vi "Assignment_01_2.vi"() -> ()   [LabVIEW 2023]
uses:
  Operations.ctl
panel:
  out "C":i64
  in  "Operations":T1
  in  "Stop":bool
  in  "N":i64
  in  "M":i64
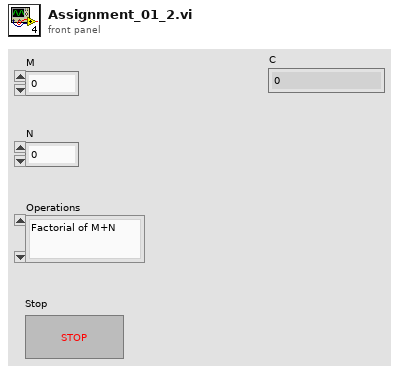
[diagram p1: front panel]
types:
  T1 = typedef "Operations.ctl" = enum16{"Factorial of M+N", "Sum of Factorial of first M Natural Numbers ", "Sum of Factorial of first N whole Numbers ", "Greater of M and N"}
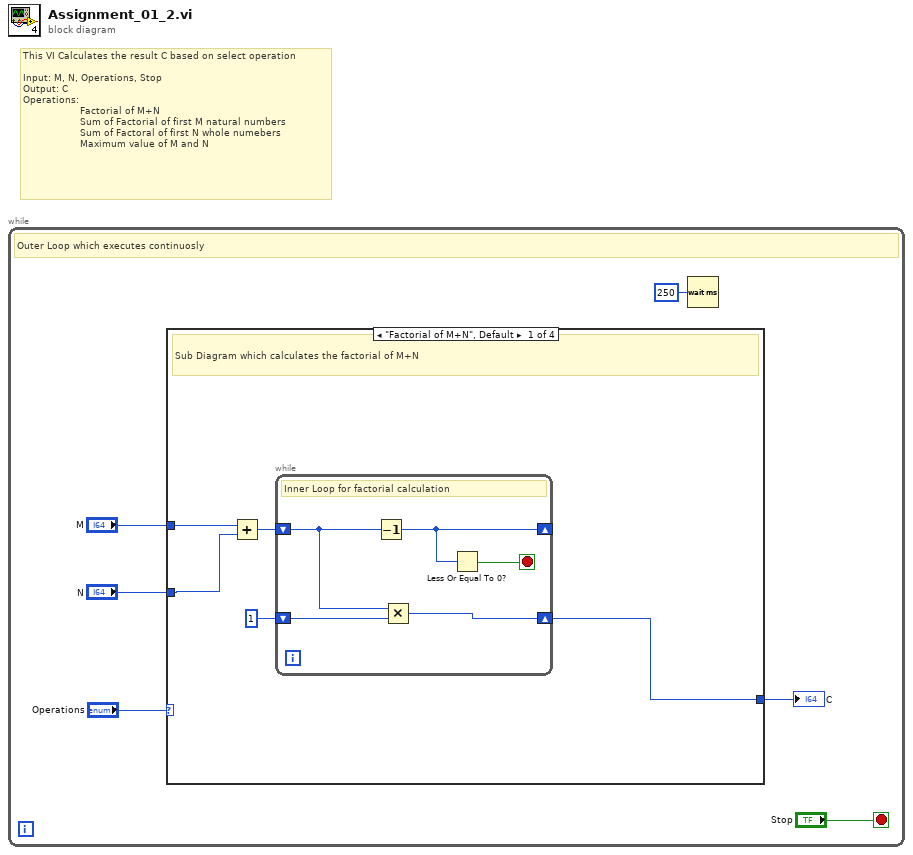
[diagram p0: block diagram]
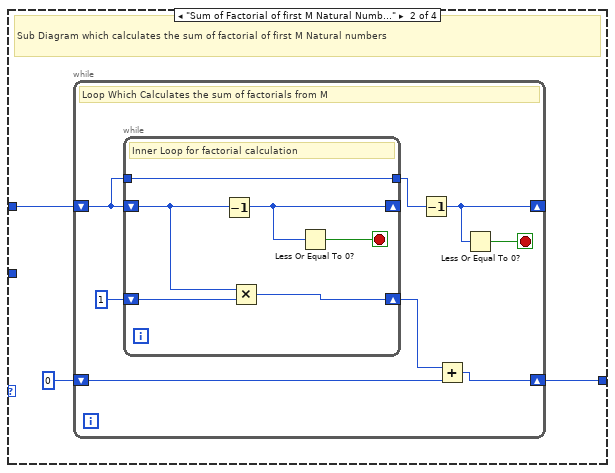
[diagram p2: hidden frame]
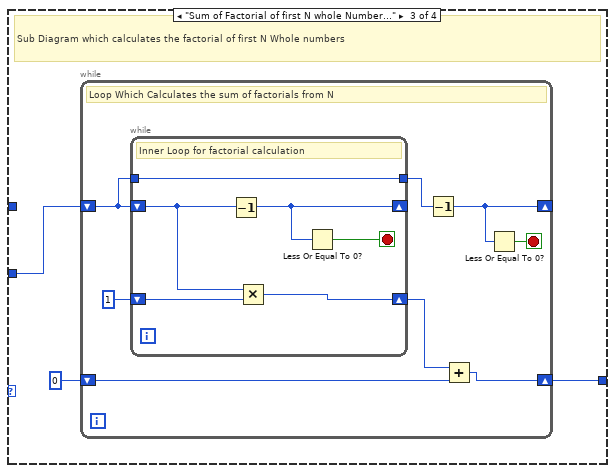
[diagram p3: hidden frame]
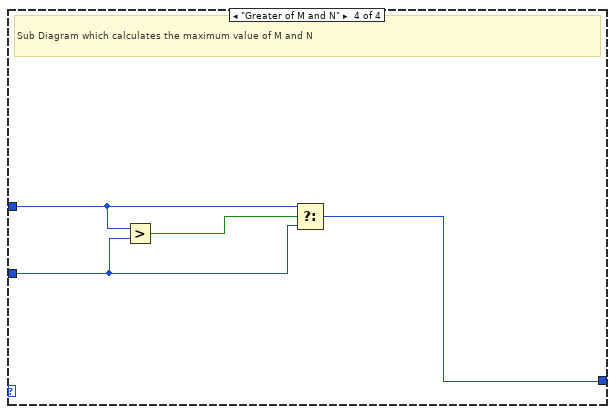
[diagram p4: hidden frame]
diagram:
  # "This VI Calculates the result C based on select operation\n\nInput: M, N, Operations, Stop\nOutput: C\nOperations:\n                   Factorial of M+N\n                   Sum of Factorial of first M natural numbers\n                   Sum of Factoral of first N whole numebers\n                   Maximum value of M and N"
  n1 = while {
    stop <- "Stop" stop-if-true
    # "Outer Loop which executes continuosly"
    n2 = case shown="\"Factorial of M+N\", Default" "Operations" {
      tunnel: "M" -> [w9 w19 _ w53]
      tunnel: "N" -> [w8 _ w35 w52]
      tunnel: [w7 w17 w34 w51] -> w3
      frame "Factorial of M+N", Default {
        # "Sub Diagram which calculates the factorial of M+N"
        n3 = Add(x=w9, y=w8) -> (x+y=w11:i64)
        n4 = while {
          shift-right: [w15] -> _
          shift-left: w11 -> [w12]
          shift-right: [w16] -> w7
          shift-left: i64 1 -> [w13]
          stop <- w14 stop-if-true
          # "Inner Loop for factorial calculation"
          n5 = Decrement(x=w12) -> (x-1=w15:i64)
          n6 = Multiply(x=w12, y=w13) -> (x*y=w16:i64)
          n7 = Less Or Equal To 0?(x=w15) -> (x <= 0?=w14:bool)
        }
      }
      frame "Sum of Factorial of first M Natural Numbers " {
        # "Sub Diagram which calculates the sum of factorial of first M Natural numbers"
        n8 = while {
          shift-right: [w25] -> _
          shift-left: w19 -> [w21]
          shift-right: [w22] -> w17
          shift-left: i64 0 -> [w24]
          stop <- w26 stop-if-true
          # "Loop Which Calculates the sum of factorials from M"
          n9 = while {
            shift-right: [w28] -> _
            shift-left: w21 -> [w31]
            shift-right: [w33] -> w23
            shift-left: i64 1 -> [w30]
            tunnel: [w29] -> w20
            tunnel: w21 -> [w29]
            stop <- w32 stop-if-true
            # "Inner Loop for factorial calculation"
            n10 = Decrement(x=w31) -> (x-1=w28:i64)
            n11 = Multiply(x=w31, y=w30) -> (x*y=w33:i64)
            n12 = Less Or Equal To 0?(x=w28) -> (x <= 0?=w32:bool)
          }
          n13 = Decrement(x=w20) -> (x-1=w25:i64)
          n14 = Add(x=w23, y=w24) -> (x+y=w22:i64)
          n15 = Less Or Equal To 0?(x=w25) -> (x <= 0?=w26:bool)
        }
      }
      frame "Sum of Factorial of first N whole Numbers " {
        # "Sub Diagram which calculates the factorial of first N Whole numbers"
        n16 = while {
          shift-right: [w42] -> _
          shift-left: w35 -> [w38]
          shift-right: [w39] -> w34
          shift-left: i64 0 -> [w41]
          stop <- w43 stop-if-true
          # "Loop Which Calculates the sum of factorials from N"
          n17 = while {
            shift-right: [w49] -> _
            shift-left: w38 -> [w47]
            shift-right: [w50] -> w40
            shift-left: i64 1 -> [w46]
            tunnel: [w45] -> w37
            tunnel: w38 -> [w45]
            stop <- w48 stop-if-true
            # "Inner Loop for factorial calculation"
            n18 = Decrement(x=w47) -> (x-1=w49:i64)
            n19 = Multiply(x=w47, y=w46) -> (x*y=w50:i64)
            n20 = Less Or Equal To 0?(x=w49) -> (x <= 0?=w48:bool)
          }
          n21 = Decrement(x=w37) -> (x-1=w42:i64)
          n22 = Add(x=w40, y=w41) -> (x+y=w39:i64)
          n23 = Less Or Equal To 0?(x=w42) -> (x <= 0?=w43:bool)
        }
      }
      frame "Greater of M and N" {
        # "Sub Diagram which calculates the maximum value of M and N"
        n24 = Greater?(x=w53, y=w52) -> (0:w54:bool)
        n25 = Select(t=w53, s=w54, f=w52) -> (s? t:f=w51:i64)
      }
    }
    "C" <- w3
    n26 = Wait (ms)(milliseconds to wait=u32 250) -> ()  [unwired: 1 out]
  }
